vi "Populate VS channel control- PWM channel by cluster.vi"(7 "DisplayFilter":u8(ring)=7 items=["K_CHAN_R", "K_CHAN_W", "K_CHAN_RW", "K_CHAN_VOLT", "K_CHAN_FAULT", "K_ALL", "K_CUSTOM", "K_CHAN_R_VIS", "K_CHAN_W_VIS", "K_CHAN_RW_VIS", "K_CHAN_VOLT_VIS", "K_CHAN_FAULT_VIS"], 8 "error in (no error)":errorcluster, 9 "Data cluster in":T1, 10 "NIVS.System Definition Root":refnum<k24>, 11 ".NET Refnum in":refnum<k24>) -> (0 "error out":errorcluster, 3 ".NET Refnum out":refnum<k24>)   [LabVIEW 2013]
uses:
  PWM Object Parameters.ctl
  NationalInstruments.VeriStand.SystemStorageUI
  NationalInstruments.VeriStand.SystemStorage
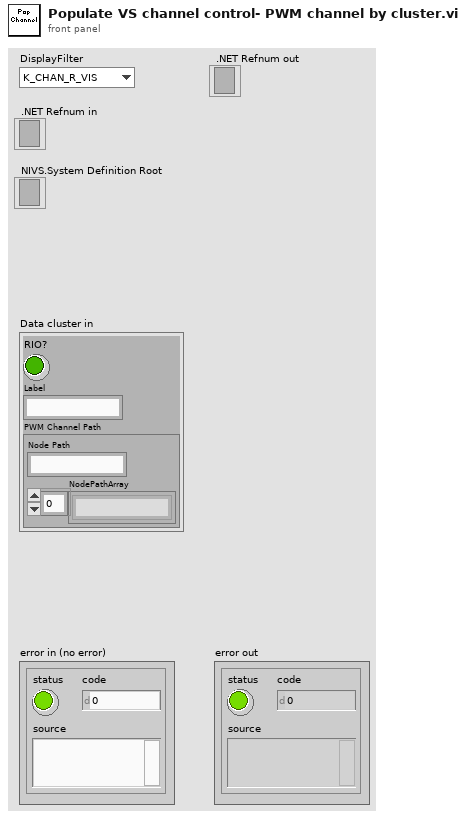
[diagram p1: front panel]
types:
  T1 = typedef "PWM Object Parameters.ctl" = cluster{"RIO?":bool, "Label":string, "PWM Channel Path":cluster{"NodePathArray":string[], "Node Path":string}}
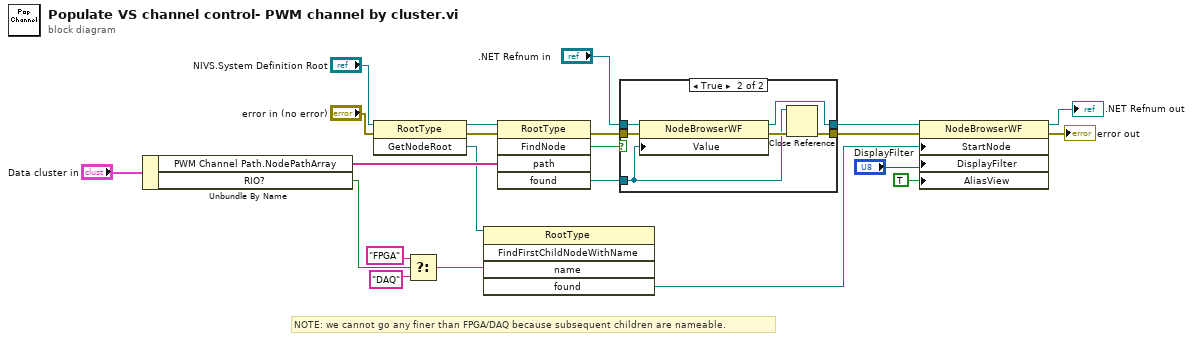
[diagram p0: block diagram]
diagram:
  # "NOTE: we cannot go any finer than FPGA/DAQ because subsequent children are nameable."
  n1 = Unbundle By Name("Data cluster in") -> ("PWM Channel Path.NodePathArray"=w3:string[], "RIO?"=w7:bool)
  n2 = invoke class="RootType" method="GetNodeRoot"(reference="NIVS.System Definition Root", error in="error in (no error)") -> (reference out=w11:refnum<k24>, error out=w10:errorcluster, "GetNodeRoot"=w2:refnum<k24>)  [unwired: 1 in]
  n3 = Select(t="FPGA", s=w7, f="DAQ") -> (s? t:f=w6:string)
  n4 = invoke class="RootType" method="FindFirstChildNodeWithName"(reference=w2, "name"=w6) -> ("found"=w1:refnum<k24>)  [unwired: 3 in, 4 out]
  n5 = invoke class="RootType" method="FindNode"(reference=w11, error in=w10, "path"=w3) -> (error out=w17:errorcluster, "FindNode"=w19:bool, "found"=w16:refnum<k24>)  [unwired: 2 in, 2 out]
  n6 = case shown="True" w19 {
    tunnel: w16 -> [_ w25]
    tunnel: w17 -> [w24 w26]
    tunnel: [w24 w29] -> w18
    tunnel: ".NET Refnum in" -> [w23 w28]
    tunnel: [w23 w27] -> w20
    frame False {
    }
    frame True {
      n7 = property class="NodeBrowserWF"(reference=w28, error in=w26, "Value"=w25) -> (reference out=w27:refnum<k24>, error out=w30:errorcluster)
      n8 = Close Reference(reference=w25, error in (no error)=w30) -> (error out=w29:errorcluster)
    }
  }
  n9 = property class="NodeBrowserWF"(reference=w20, error in=w18, "StartNode"=w1, "DisplayFilter"="DisplayFilter", "AliasView"=TRUE) -> (reference out=→".NET Refnum out":refnum<k24>, error out=→"error out":errorcluster)
